vi "GetStatus.vi"(8 "error in (no error)":errorcluster, 11 "Device in":refnum<class "Device.lvclass">) -> (0 "error out":errorcluster, 2 "Status":T1 items=["Offline", "Idle", "Busy"], 3 "Device out":refnum<class "Device.lvclass">)   [LabVIEW 2020, in "Device.lvlib" / "Device.lvclass"]
uses:
  Device.lvclass
  DeviceStatus.ctl
  Device.lvclass/Device.ctl
  Device.lvlib
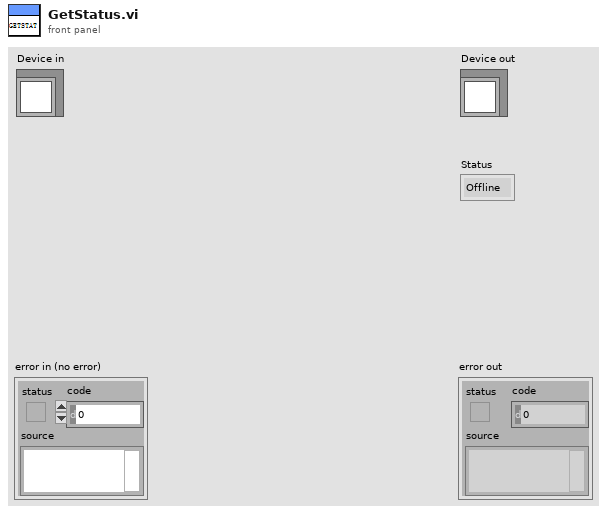
[diagram p1: front panel]
types:
  T1 = typedef "Device.lvlib/DeviceStatus.ctl" = i32
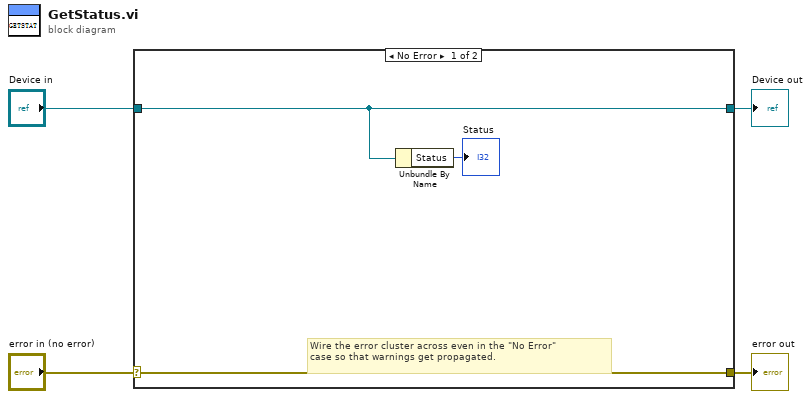
[diagram p0: block diagram]
diagram:
  n1 = case shown="No Error" "error in (no error)" {
    selector: "error in (no error)" -> [w7 w9]
    tunnel: [w7 w9] -> w3
    tunnel: [w6 w8] -> w1
    tunnel: "Device in" -> [w6 w8]
    frame No Error {
      # "Wire the error cluster across even in the \"No Error\"\ncase so that warnings get propagated."
      n2 = Unbundle By Name(w6) -> ("Status"=→"Status":T1)
    }
    frame Error {
    }
  }
  "error out" <- w3
  "Device out" <- w1
